vi "ReadEyeFileFast_Poly.vi"   [LabVIEW 2022 SP3]
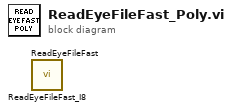
[diagram p0: block diagram]
diagram:
  n1 = call "ReadEyeFileFast_I8.vi"() -> ()  [unwired: 9 in, 11 out]
  n2 = call "ReadEyeFileFast.vi"() -> ()  [unwired: 14 in, 6 out]
